vi "Demo-Browse2.vi"() -> ()   [LabVIEW 2017]
uses:
  opcua-lvlib/TypeDefs/Data Type.ctl
  opcua-lvlib/Browser/Server Classes/UA Server/UA Server.lvclass
  C:/Users/108003658/OneDrive - Baker Hughes/Desktop/opcua-0_2_0/opcua-lvlib/Browser/Server Classes/Base Tree/Base Tree.lvclass
  opcua-lvlib/Server/Server.lvclass
  opcua-lvlib/opcua.lvlib
  opcua-lvlib/Client/Client.lvclass
  opcua-lvlib/Browser/Server Classes/Base Tree/Base Tree.lvclass
panel:
  out "selected":string
  out "My Sine Value":dbl
  out "Node Info":string
  out "# Nodes":i32
  in  "Tree":string(tree)
  out "MyVariable (Client)":i32
  out "My Variable (Server)":i32
  in  "Stop Button":bool
  # "Warning!  Please use the Stop Button at all times and not Abort Execution by LabVIEW. \nOtherwise, the handles will not be closed, and you will get an Exception next time. \nThis is because Process Detach/Thread Detach are not handled yet. Gets changed later."
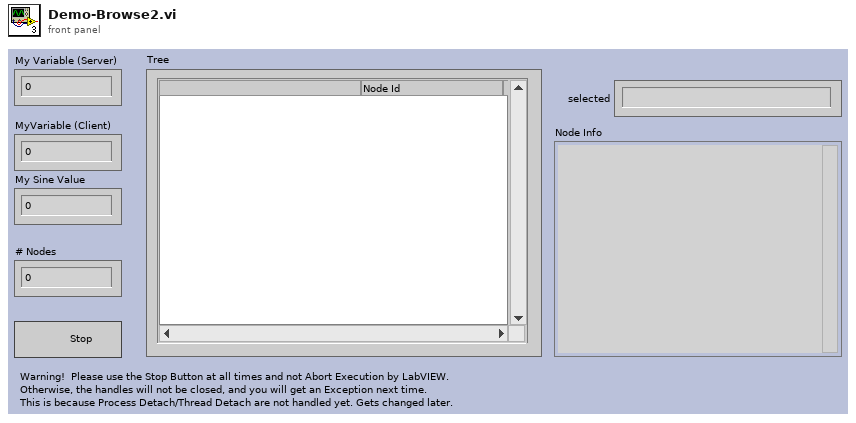
[diagram p1: front panel]
types:
  T1 = typedef "opcua.lvlib/Data Type.ctl" = u16
  T2 = enum32{"invalid app kind", "Development System", "Run Time System", "Student Edition", "Embedded LabVIEW", "Evaluation", "Custom"}
  T3 = typedef "opcua.lvlib/Node.ctl" = cluster{"class":i32, "Display Name":string, "Node UID":string}
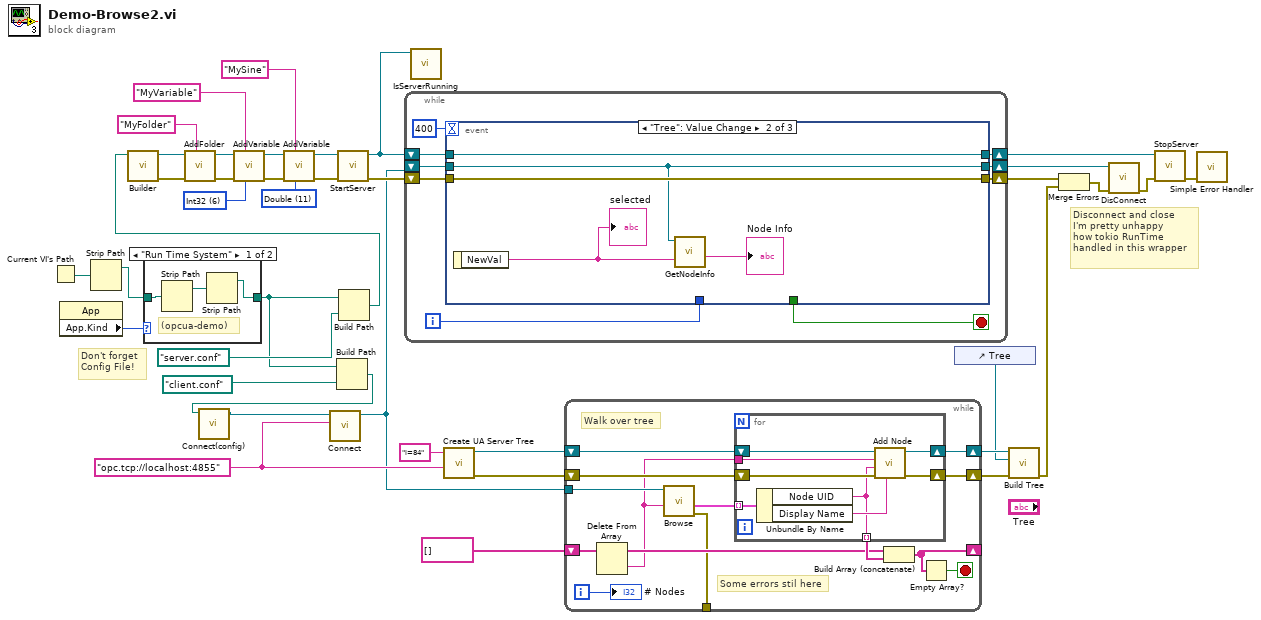
[diagram p0: block diagram]
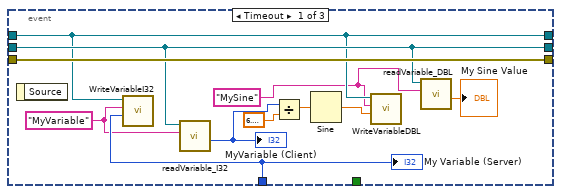
[diagram p3: hidden frame]
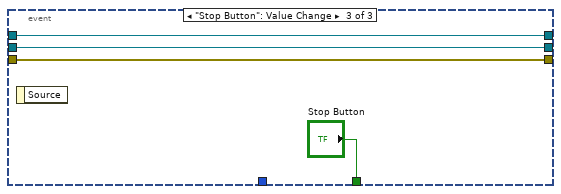
[diagram p4: hidden frame]
diagram:
  w1 = T1 11 items=["Boolean"=1, "SByte"=2, "Byte"=3, "Int16"=4, "UInt16"=5, "Int32"=6, "UInt32"=7, "Int64"=8, "UInt64"=9, "Float"=10, "Double"=11, "String"=12, "DateTime"=13, "ByteString"=15, "Array of Boolean"=101, "Array of SByte"=102, "Array of Byte"=103, "Array of Int16"=104, "Array of UInt16"=105, "Array of Int32"=106, "Array of UInt32"=107, "Array of Int64"=108, "Array of UInt64"=109, "Array of Float"=110, "Array of Double"=111, "Array of String"=112, "Array of DateTime"=113, "Array of ByteString"=115, "Matrix of Boolean"=201, "Matrix of SByte"=202, "Matrix of Byte"=203, "Matrix of Int16"=204, "Matrix of UInt16"=205, "Matrix of Int32"=206, "Matrix of UInt32"=207, "Matrix of Int64"=208, "Matrix of UInt64"=209, "Matrix of Float"=210, "Matrix of Double"=211, "Matrix of String "=212, "Matrix of DateTime"=213, "Matrix of ByteString"=215] ("type")
  w24 = "opc.tcp://localhost:4855" ("URL")
  w34 = T1 6 items=["Boolean"=1, "SByte"=2, "Byte"=3, "Int16"=4, "UInt16"=5, "Int32"=6, "UInt32"=7, "Int64"=8, "UInt64"=9, "Float"=10, "Double"=11, "String"=12, "DateTime"=13, "ByteString"=15, "Array of Boolean"=101, "Array of SByte"=102, "Array of Byte"=103, "Array of Int16"=104, "Array of UInt16"=105, "Array of Int32"=106, "Array of UInt32"=107, "Array of Int64"=108, "Array of UInt64"=109, "Array of Float"=110, "Array of Double"=111, "Array of String"=112, "Array of DateTime"=113, "Array of ByteString"=115, "Matrix of Boolean"=201, "Matrix of SByte"=202, "Matrix of Byte"=203, "Matrix of Int16"=204, "Matrix of UInt16"=205, "Matrix of Int32"=206, "Matrix of UInt32"=207, "Matrix of Int64"=208, "Matrix of UInt64"=209, "Matrix of Float"=210, "Matrix of Double"=211, "Matrix of String "=212, "Matrix of DateTime"=213, "Matrix of ByteString"=215] ("type")
  # "Disconnect and close\nI'm pretty unhappy\nhow tokio RunTime\nhandled in this wrapper"
  # "Don't forget\nConfig File!"
  n1 = Current VI's Path() -> (path=w37:path)
  n2 = property class="App"() -> ("App.Kind"=w13:T2)  [unwired: 2 in, 2 out]
  n3 = Strip Path(path=w37) -> (stripped path=w12:path)  [unwired: 1 out]
  n4 = case shown="\"Run Time System\"" w13 {
    tunnel: w12 -> [w43 w44]
    tunnel: [w41 w44] -> w7
    frame "Run Time System" {
      # "(opcua-demo)"
      n5 = Strip Path(path=w43) -> (stripped path=w42:path)  [unwired: 1 out]
      n6 = Strip Path(path=w42) -> (stripped path=w41:path)  [unwired: 1 out]
    }
    frame "Development System", Default {
    }
  }
  n7 = Build Path(base path=w7, name or relative path=path "client.conf" ("Config File Path")) -> (appended path=w8:path)
  n8 = call "Connect(config).vi"("path to client config"=w8) -> ("Client out"=w9:refnum<class "Client.lvclass">)  [unwired: 9 in, 1 out]
  n9 = call "Connect.vi"("URL"=w24, "Client In"=w9) -> ("Client out"=w16:refnum<class "Client.lvclass">)  [unwired: 7 in, 2 out]
  n10 = Build Path(base path=w7, name or relative path=path "server.conf" ("Config File Path")) -> (appended path=w11:path)
  n11 = call "Builder.vi"("Config File Path"=w11) -> ("error out"=w39:errorcluster, "Server out"=w40:refnum<class "Server.lvclass">)  [unwired: 8 in, 1 out]
  n12 = call-dynamic "AddFolder.vi"("folder_node"="MyFolder", "error in (no error)"=w39, "Server in"=w40) -> ("error out"=w32:errorcluster, "Server out"=w33:refnum<class "Server.lvclass">)  [unwired: 7 in]
  n13 = call-dynamic "AddVariable.vi"("type"=w34, "variable_node"="MyVariable" ("folder_node"), "error in (no error)"=w32, "Server in"=w33) -> ("error out"=w4:errorcluster, "Server out"=w6:refnum<class "Server.lvclass">)  [unwired: 6 in]
  n14 = call-dynamic "AddVariable.vi"("type"=w1, "variable_node"="MySine" ("folder_node"), "error in (no error)"=w4, "Server in"=w6) -> ("error out"=w3:errorcluster, "Server out"=w5:refnum<class "Server.lvclass">)  [unwired: 6 in]
  n15 = call-dynamic "StartServer.vi"("error in (no error)"=w3, "Server in"=w5) -> ("error out"=w28:errorcluster, "Server out"=w30:refnum<class "Server.lvclass">)  [unwired: 8 in]
  n16 = while {
    shift-right: [w49] -> w31
    shift-left: w30 -> [w52]
    shift-right: [w48] -> w27
    shift-left: w28 -> [w47]
    shift-right: [w46] -> w15
    shift-left: w16 -> [w45]
    i -> [w51]
    stop <- w50 stop-if-true
    n17 = event shown="[1] \"Tree\": Value Change" {
      selector: _ -> [_ _ _]
      dyn-events: _ -> [_ _ _]
      timeout: 400 -> [_ _ _]
      tunnel: w52 -> [w56 w69 w72]
      tunnel: w51 -> [w63 _ _]
      tunnel: [_ _ "Stop Button"] -> w50
      tunnel: [w56 w69 w72] -> w49
      tunnel: [w64 w68 w71] -> w48
      tunnel: w47 -> [w64 w68 w71]
      tunnel: [w58 w65 w70] -> w46
      tunnel: w45 -> [w58 w65 w70]
      event Timeout {
        w55 = "MySine" ("variable_node")
        w62 = "MyVariable" ("folder_node")
        n18 = event-data() -> ()  [unwired: 1 in, 1 out]
        n19 = call-dynamic "WriteVariableI32.vi"("value"=w63, "variable_node"=w62, "Server in"=w56) -> ()  [unwired: 7 in, 2 out]
        n20 = call "readVariable_I32.vi"("URL"=w62, "Client In"=w58) -> ("val"=w61:i32)  [unwired: 6 in, 3 out]
        "MyVariable (Client)" <- w61
        n21 = Divide(x=w61, y=6.283185307179586) -> (x/y=w59:dbl)
        n22 = Sine(x=w59) -> (sin(x)=w54:dbl)
        n23 = call-dynamic "WriteVariableDBL.vi"("value"=w54, "variable_node"=w55, "Server in"=w56) -> ()  [unwired: 7 in, 2 out]
        n24 = call "readVariable_DBL.vi"("URL"=w55, "Client In"=w58) -> ("val"=→"My Sine Value":dbl)  [unwired: 6 in, 3 out]
        "My Variable (Server)" <- w63
      }
      event "Tree": Value Change {
        n25 = event-data() -> ("NewVal"=w66:string)  [unwired: 1 in]
        "selected" <- w66
        n26 = call "GetNodeInfo.vi"("id as String"=w66, "Client In"=w65) -> ("Node Info"=→"Node Info":string)  [unwired: 6 in, 3 out]
      }
      event "Stop Button": Value Change {
        n27 = event-data() -> ()  [unwired: 1 in, 1 out]
      }
    }
  }
  n28 = call-dynamic "IsServerRunning.vi"("Server in"=w30) -> ()  [unwired: 8 in, 3 out]
  n29 = call "Create UA Server Tree.vi"("Display Name"=w24, "Server Endpoint URL (Root folder)"="i=84" ("Display Name")) -> ("Error Out"=w19:errorcluster, "UA Server Tree"=w20:refnum<class "UA Server.lvclass">)  [unwired: 8 in]
  n30 = while {
    shift-right: [w83] -> w23
    shift-left: w20 -> [w87]
    shift-right: [w85] -> _
    shift-left: string[] [] -> [w82]
    tunnel: w16 -> [w78]
    shift-right: [w79] -> w21
    shift-left: w19 -> [w80]
    tunnel: [w75] -> _
    i -> [w76]
    stop <- w84 stop-if-true
    # "Some errors stil here"
    # "Walk over tree"
    n31 = Delete From Array(array=w82) -> (deleted portion=w74:string, array with subset deleted=w81:string[])  [unwired: 2 in]
    n32 = call "Browse.vi"("id as String"=w74, "Client In"=w78) -> ("error out"=w75:errorcluster, "result"=w77:T3[])  [unwired: 6 in, 2 out]
    n33 = for {
      tunnel: w77 -> [w94] mode=indexing
      tunnel: w74 -> [w89]
      tunnel: [w88] -> w86 mode=indexing
      shift-right: [w93] -> w83
      shift-left: w87 -> [w95]
      shift-right: [w91] -> w79
      shift-left: w80 -> [w92]
      n34 = Unbundle By Name(w94) -> ("Node UID"=w88:string, "Display Name"=w90:string)
      n35 = call-dynamic "Add Node.vi"("Display Name"=w90, "error in (no error)"=w92, "UID"=w88, "Parent"=w89, "Base Tree in"=w95) -> ("error out"=w91:errorcluster, "Base Tree out"=w93:refnum<class "UA Server.lvclass">)  [unwired: 5 in]
    }
    n36 = Build Array (concatenate)(w81, w86) -> (w85:string[])
    n37 = Empty Array?(array=w85) -> (empty?=w84:bool)
    "# Nodes" <- w76
  }
  n38 = control-ref of="Tree"() -> (w18:refnum<vi>)
  n39 = call "Build Tree.vi"("error in (no error)"=w21, "Tree Reference"=w18, "Base Tree in"=w23) -> ("error out"=w14:errorcluster)  [unwired: 7 in, 1 out]
  n40 = Merge Errors(w27, w14) -> (w26:errorcluster)
  n41 = call "DisConnect.vi"("error in (no error)"=w26, "Client In"=w15) -> ("error out"=w29:errorcluster)  [unwired: 7 in, 2 out]
  n42 = call-dynamic "StopServer.vi"("error in (no error)"=w29, "Server in"=w31) -> ("error out"=w25:errorcluster)  [unwired: 7 in, 2 out]
  n43 = call <vilib>:"Simple Error Handler.vi"("error in (no error)"=w25) -> ()  [unwired: 4 in, 5 out]
